vi "deleteFiles.vi"   [LabVIEW 2017]
doc: "Checks if any frame has been saved. If not, it deletes the whole folder to remove the clutter."
uses:
  globalUtilities.vi
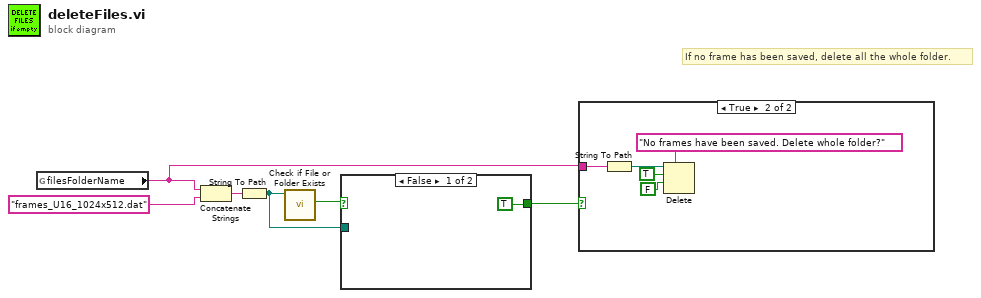
[diagram p0: block diagram]
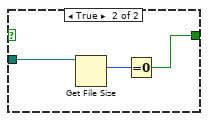
[diagram p2: hidden frame]
diagram:
  # "If no frame has been saved, delete all the whole folder."
  n1 = global read "globalUtilities.vi" "filesFolderName"() -> (w4:string)
  n2 = Concatenate Strings(w4, "frames_U16_1024x512.dat") -> (w5:string)
  n3 = String To Path(string=w5) -> (path=w1:path)
  n4 = call <vilib>:"Check if File or Folder Exists.vi"("path"=w1) -> ("file or folder exists?"=w2:bool)  [unwired: 8 in, 2 out]
  n5 = case shown="False" w2 {
    tunnel: [TRUE w9] -> w3
    tunnel: w1 -> [_ w8]
    frame False {
    }
    frame True {
      n6 = Get File Size(file=w8) -> (size (in bytes)=w10:i64)  [unwired: 1 in, 2 out]
      n7 = Equal To 0?(x=w10) -> (x = 0?=w9:bool)
    }
  }
  n8 = case shown="True" w3 {
    tunnel: w4 -> [_ w15]
    frame False {
    }
    frame True {
      n9 = String To Path(string=w15) -> (path=w14:path)
      n10 = Delete(prompt (Delete)="No frames have been saved. Delete whole folder?", path (use dialog)=w14, entire hierarchy (F)=TRUE, confirm (F)=FALSE) -> ()  [unwired: 1 in, 3 out]
    }
  }
